vi "Phasor Convert z or (g,s) to g & s.vi"(9 "Phasor":T1={"g"=nan, "s"=nan}, 11 "z":cdb=nan+nani) -> (1 "s":dbl, 3 "g":dbl)   [LabVIEW 2021, in "Phasor.lvlib"]
uses:
  Phasor.lvlib
  Phasor (g, s).ctl
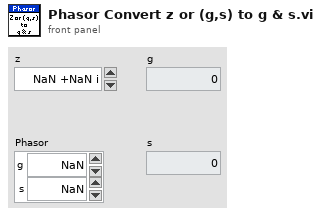
[diagram p1: front panel]
types:
  T1 = typedef "Phasor.lvlib/Phasor (g, s).ctl" = cluster{"g":dbl, "s":dbl}
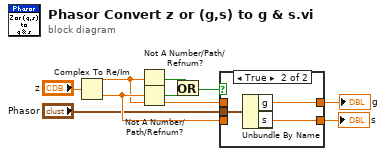
[diagram p0: block diagram]
diagram:
  n1 = Complex To Re/Im(x + iy="z") -> (x=w8:dbl, y=w9:dbl)
  n2 = Not A Number/Path/Refnum?(number/path/refnum=w8) -> (NaN/Path/Refnum?=w4:bool)
  n3 = Not A Number/Path/Refnum?(number/path/refnum=w9) -> (NaN/Path/Refnum?=w7:bool)
  n4 = Or(x=w4, y=w7) -> (x .or. y?=w6:bool)
  n5 = case shown="True" w6 {
    tunnel: "Phasor" -> [_ w14]
    tunnel: [w11 w13] -> w2
    tunnel: [w10 w12] -> w3
    tunnel: w8 -> [w11 _]
    tunnel: w9 -> [w10 _]
    frame False {
    }
    frame True {
      n6 = Unbundle By Name(w14) -> ("g"=w13:dbl, "s"=w12:dbl)
    }
  }
  "s" <- w3
  "g" <- w2
